vi "Format Metadata.vi"(0 "Channel in":refnum<class "Channel.lvclass">, 7 "Prefix":string, 11 "error in (no error)":errorcluster) -> (4 "Channel out":refnum<class "Channel.lvclass">, 8 "String":string, 15 "error out":errorcluster)   [LabVIEW 2015, in "Channel.lvclass"]
uses:
  Channel.lvclass
  Waveforms/Waveform/Waveform.lvclass
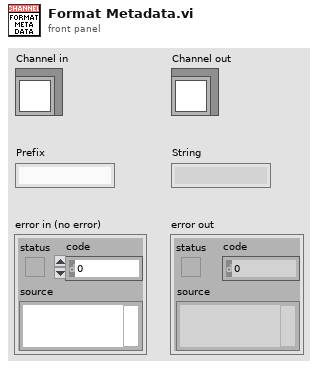
[diagram p1: front panel]
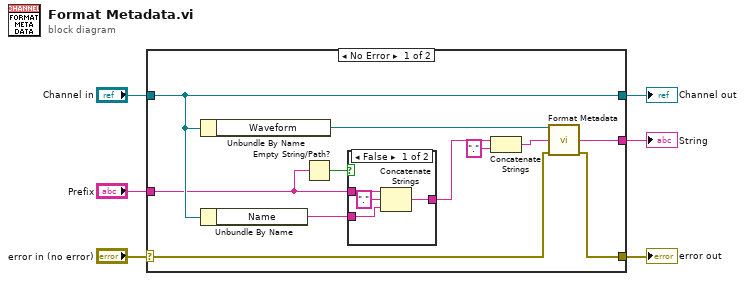
[diagram p0: block diagram]
diagram:
  n1 = case shown="No Error" "error in (no error)" {
    selector: "error in (no error)" -> [w16 w24]
    tunnel: [w15 w24] -> w5
    tunnel: [w12 w23] -> w3
    tunnel: "Channel in" -> [w12 w23]
    tunnel: "Prefix" -> [w7 _]
    tunnel: [w14 _] -> w1
    frame No Error {
      n2 = Unbundle By Name(w12) -> ("Waveform"=w17:refnum<class "Waveform.lvclass">)
      n3 = Unbundle By Name(w12) -> ("Name"=w11:string)
      n4 = Empty String/Path?(string/path=w7) -> (empty?=w13:bool)
      n5 = case shown="False" w13 {
        tunnel: w11 -> [w18 w22]
        tunnel: [w20 w22] -> w10
        tunnel: w7 -> [w21 _]
        frame False {
          n6 = Concatenate Strings(w21, "." ("string"), w18) -> (w20:string)
        }
        frame True {
        }
      }
      n7 = Concatenate Strings(w10, "." ("string")) -> (w9:string)
      n8 = call-dynamic "Format Metadata.vi"("Waveform in"=w17, "Prefix"=w9, "error in (no error)"=w16) -> ("String"=w14:string, "error out"=w15:errorcluster)  [unwired: 10 in, 1 out]
    }
    frame Error {
    }
  }
  "error out" <- w5
  "Channel out" <- w3
  "String" <- w1
